vi "Command-Line Get Numeric Key.vi"(4 "numeric key":string) -> (0 "key found?":bool, 2 "numeric value":dbl)   [LabVIEW 2015]
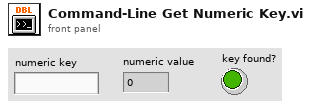
[diagram p1: front panel]
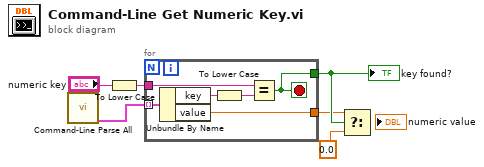
[diagram p0: block diagram]
diagram:
  n1 = call "Command-Line Parse All.vi"() -> ("numeric keys"=w1:cluster{"key":string, "value":dbl}[])  [unwired: 6 in, 5 out]
  n2 = To Lower Case(string="numeric key") -> (all lower case string=w6:string)
  n3 = for {
    tunnel: w1 -> [w12] mode=indexing
    tunnel: w6 -> [w9]
    tunnel: [w8] -> w4
    tunnel: [w7] -> w3
    stop <- w8 stop-if-true
    n4 = Unbundle By Name(w12) -> ("key"=w11:string, "value"=w7:dbl)
    n5 = To Lower Case(string=w11) -> (all lower case string=w10:string)
    n6 = Equal?(x=w9, y=w10) -> (x = y?=w8:bool)
  }
  "key found?" <- w4
  n7 = Select(t=w3, s=w4, f=0.0) -> ()  [unwired: 1 out]
